vi "HTMLPlot_Create.vi"(0 "reference in":refnum<class "HTMLPlot.lvclass">, 1 "GraphContainer":refnum<k7>, 5 "error in (no error)":errorcluster, 6 "PlotType":T1) -> (14 "reference out":refnum<class "HTMLPlot.lvclass">, 19 "error out":errorcluster)   [LabVIEW 2019, in "HTMLPlot.lvclass"]
uses:
  HTMLPlot.lvclass
  <vilib>/numeric/Random Number (Range) U64.vi
  Controls/PlotType.ctl
panel:
  out "ReadyState":i32(ring)=4 items=["READYSTATE_UNINITIALIZED", "READYSTATE_LOADING", "READYSTATE_LOADED", "READYSTATE_INTERACTIVE", "READYSTATE_COMPLETE"]
  out "Get Reqest":string
  out "concatenated string":string
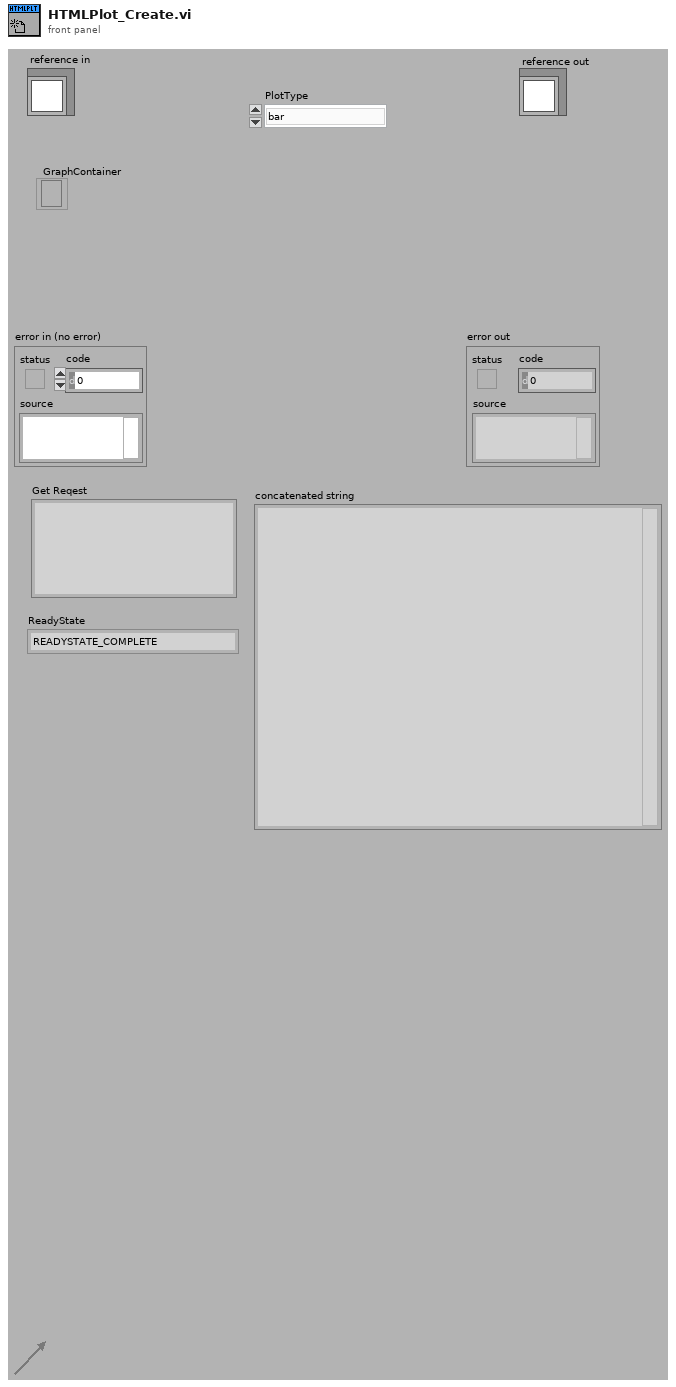
[diagram p1: front panel]
types:
  T1 = typedef "HTMLPlot.lvclass/PlotType.ctl" = enum16{"bar", "line", "pie"}
  T2 = enum16{"Standard", "Buffered", "CRLF", "Immediate"}
  T3 = typedef "HTMLPlot.lvclass/ObjectAttributes.ctl" = cluster{"Attribute1":dbl, "GraphContainer":refnum<k7>, "ChartScriptFile":string, "UtilScriptFile(demoData)":string, "BaseHTML":string, "GenericProperties":cluster{"PlotType":T1, "PlotTitle":string, "XLabel":string, "YLabel":string, "ShowToolTip":bool}, "LegendProperties":cluster{"Show":bool, "Position":T4}, "BarPlot":cluster{"Dataset":dbl[][], "DatasetLabels":string[], "XLabels":string[], "PlotColours":u32[], "Stacked":bool}, "PiePlot":cluster{"Dataset":dbl[][], "DatasetLabels":string[], "PlotColours":u32[], "DoughnutStyle":bool, "PlotLabels":string[]}, "connection ID":refnum<k5>, "PortID":u64}
  T4 = typedef "HTMLPlot.lvclass/LegendPosition.ctl" = enum16{"top", "right", "left", "bottom"}
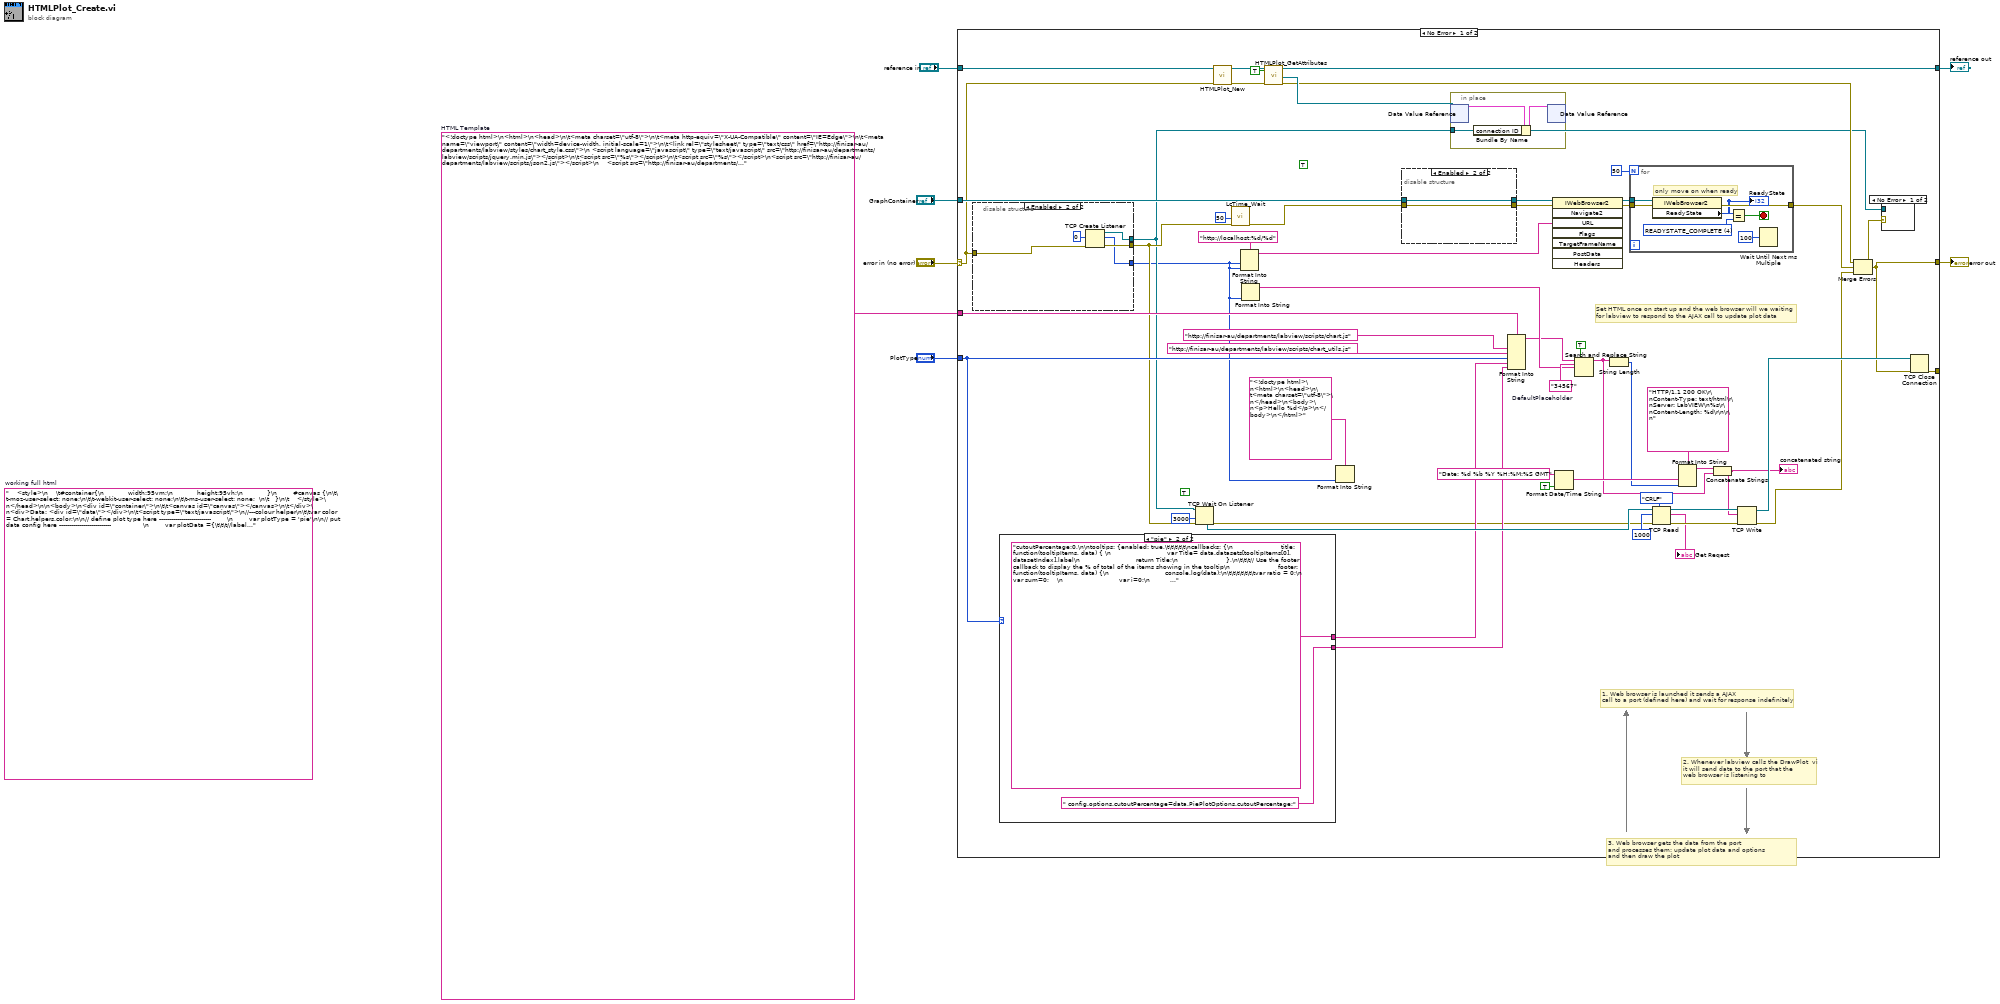
[diagram p0: block diagram]
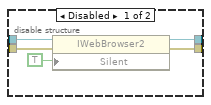
[diagram p2: hidden frame]
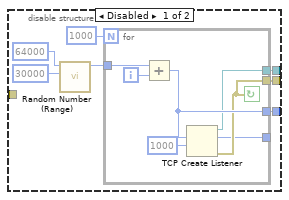
[diagram p3: hidden frame]
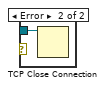
[diagram p4: hidden frame]
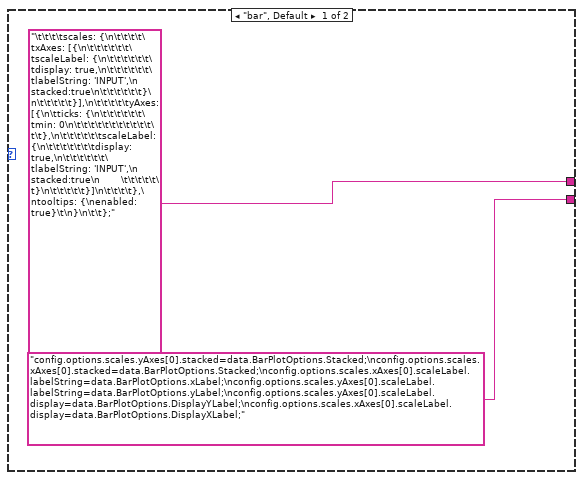
[diagram p5: hidden frame]
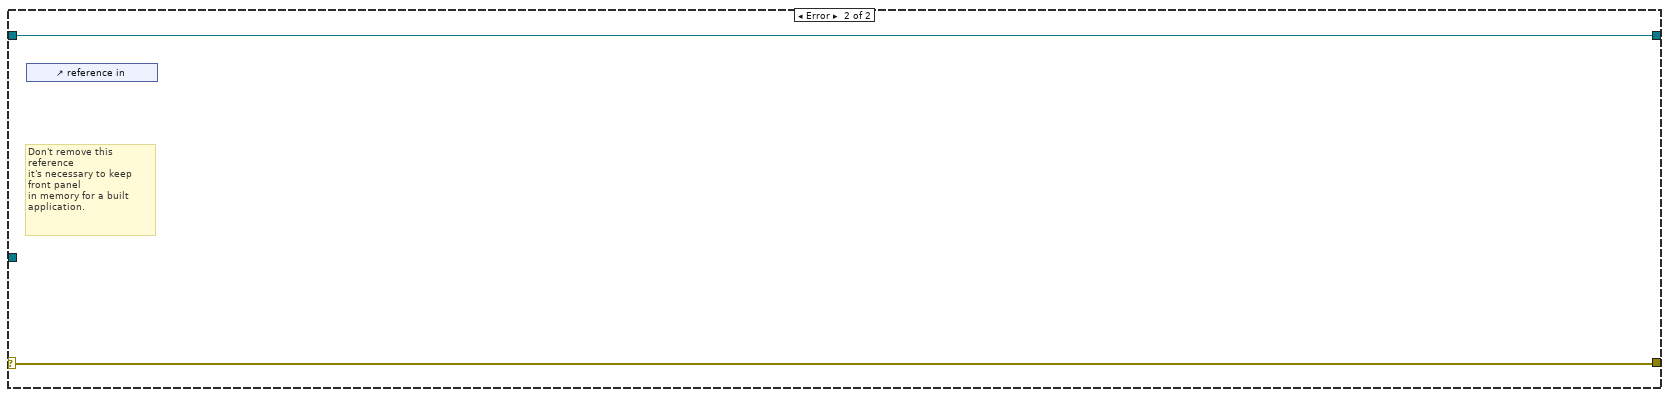
[diagram p6: hidden frame]
diagram:
  (unwired) "    <style>\n    \t#container{\n            width:95vm;\n            height:95vh;\n            }\n        #canvas {\n\t\t-moz-user-select: none;\n\t\t-webkit-user-select: none;\n\t\t-ms-user-select: none;  \n\t   }\n\t    </style>\n</head>\n\n<body>\n<div id=\"container\">\n\t\t<canvas id=\"canvas\"></canvas>\n\t</div>\n<div>Data: <div id=\"data\"></div>\n\t<script type=\"text/javascript\">\n//---colour helper\n\t\tvar color = Chart.helpers.color;\n\n// define plot type here --------------------------        \n        var plotType = 'pie'\n\n// put data config here --------------------------                \n        var plotData ={\t\t\t//labels\n   \tlabels: ['DLP2','SLP','DWP','DLP3'\n],\n    //datasets\n   datasets:[{\n\t\t\t\tlabel: 'Q1',\n\t\t\t\tbackgroundColor: ['#5C8260','#FF88C2','#2400B4','#FFF242'\n],\n\t\t\t\tdata: [3.000000,5.000000,7.000000,89.000000\n]\n\t\t\t},{\n\t\t\t\tlabel: 'Q2',\n\t\t\t\tbackgroundColor: ['#5C8260','#FF88C2','#2400B4','#FFF242'\n],\n\t\t\t\tdata: [2.000000,9.000000,3.000000,6.000000\n]\n\t\t\t}]}   \n// put plot options here --------------------------\n        var plotOptions ={responsive: true,\nmaintainAspectRatio: false,\n\t\t\t\tanimation: {\n\t\t\t\t\tanimateScale: true,\n\t\t\t\t\tanimateRotate: true\n\t\t\t\t},\nlegend: {\ndisplay:true,\t\t\t\t\t\t\nposition: 'right'\n\t\t\t\t\t},title: {\n\t\t\t\t\t\tdisplay:true,\n\t\t\t\t\t\ttext: 'Prouduction Summary 2020'\n\t\t\t\t\t}, tooltips: {enabled: true,\t\t\t\t\tcallbacks: {\n                        title: function(tooltipItems, data) { \n                            //console.log(data);\n                        var Title= data.datasets[tooltipItems[0].datasetIndex].label\n                            return Title;\n                        },\n\t\t\t// Use the footer callback to display the % of total of the items showing in the tooltip\n                        footer: function(tooltipItems, data) {\n                            console.log(data);\n\t\t\t\t\t\t\tvar ratio = 0;\n                            var sum=0;    \n                            var i=0;\n                            var length = data.datasets[tooltipItems[0].datasetIndex].data.length;\n                            for( i=0;i<length;i++){\n                                sum+= data.datasets[tooltipItems[0].datasetIndex].data[i];\n                            }\n\t\t\t\t\t\t\ttooltipItems.forEach(function(tooltipItem) {\n\t\t\t\t\t\t\t\tratio = 100*data.datasets[tooltipItem.datasetIndex].data[tooltipItem.index]/sum;\n                                ratio=ratio.toFixed(1)\n\t\t\t\t\t\t\t});\n\t\t\t\t\t\t\treturn 'ratio: ' + ratio + '%' ;\n\t\t\t\t\t\t},\n\t\t\t\t\t},\n\t\t\t\t\tfooterFontStyle: 'normal'}\t}\n // summarise config here --------------------------                   \n        var config = {\n\t\t\ttype: plotType,\n\t\t\tdata: plotData,\n\t\t\toptions: plotOptions\n\t\t};\n\n// run plot function here -------------------------- \n        \n\t\twindow.onload = function() {\n\t\t\tvar ctx = document.getElementById('canvas').getContext('2d');\n\t\t\twindow.myChart = new Chart(ctx, config); \n   CheckForEvents();\n\t\t};\n\nfunction CheckForEvents() {        \n        $.ajax({\n            url:'http://localhost:34567/action',\n             method:'GET',\n             dataType:'json',\n       \n            success: function(data){\n            config.type=data.data.PlotType;\n $(\"#data\").text(data.data.PlotData);\n console.log(data.data.PlotData);\nvar myObj = JSON.parse(data.data.PlotData);\n            config.data=myObj;\n console.log(myObj);\n//config.options=data.data.Options;\n          \n          window.myChart.update(); \n            CheckForEvents();\n            }\n        })\n     }\n\t</script>\n</body>\n</html>"  # working full html
  w2 = "<!doctype html>\n<html>\n<head>\n\t<meta charset=\"utf-8\">\n\t<meta http-equiv=\"X-UA-Compatible\" content=\"IE=Edge\">\n\t<meta name=\"viewport\" content=\"width=device-width, initial-scale=1\">\n\t<link rel=\"stylesheet\" type=\"text/css\" href=\"http://finisar-au/departments/labview/styles/chart_style.css\">\n <script language=\"javascript\" type=\"text/javascript\" src=\"http://finisar-au/departments/labview/scripts/jquery.min.js\"></script>\n\t<script src=\"%s\"></script>\n\t<script src=\"%s\"></script>\n<script src=\"http://finisar-au/departments/labview/scripts/json2.js\"></script>\n    <script src=\"http://finisar-au/departments/labview/scripts/jquery(v1.11.3).min.js\"></script>\n    <style>\n    \t#container{\n            width:95vm;\n            height:95vh;\n            }\n        #canvas {\n\t\t-moz-user-select: none;\n\t\t-webkit-user-select: none;\n\t\t-ms-user-select: none;  \n\t   }\n\t    </style>\n</head>\n\n<body>\n<div id=\"container\">\n\t\t<canvas id=\"canvas\"></canvas>\n\t</div>\n\t<script type=\"text/javascript\">\n//---colour helper\nvar color = Chart.helpers.color;\nvar plotData ={}  \n\n // summarise config here --------------------------                   \n        var config = {\n\n// **************** PLOT TYPE***************************\n\t\t\ttype: '%s',\n\n\t\t\tdata: plotData,\n//\t\t\t **************** PLOT OPTIONS : THIS PART WILL BE PLOT TYPE DEPENDENT***************************\noptions: \n{\nresponsive: true,\nmaintainAspectRatio: false,\n\t\t\t\tanimation: {\n\t\t\t\t\tanimateScale: true,\n\t\t\t\t\tanimateRotate: true\n\t\t\t\t},\nlegend: {\ndisplay:false,\t\t\t\t\t\t\nposition: 'right'\n\t\t\t\t\t},\ntitle: {\n\t\t\t\t\t\tdisplay:true,\n\t\t\t\t\t\ttext: 'INPUT'\n\t\t\t\t\t},  \n//*************************  ADDITIONAL OPTIONS   ***********************\n%s\n\n// run plot function here -------------------------- \n        \n\t\twindow.onload = function() {\n\t  var ctx = document.getElementById('canvas').getContext('2d');\n\t\t\twindow.myChart = new Chart(ctx, config); \n   CheckForEvents();\n\t\t};\n\nfunction CheckForEvents() {        \n        $.ajax({\n            url:'http://localhost:34567/action',\n             method:'GET',\n             dataType:'json',\n       \n            success: function(data){\n            var myData = JSON.parse(data.PlotData);\n            config.data=myData;\n\n            config.options.legend.display= data.GenericPlotOptions.LegendDisplay;\n            config.options.legend.position=data.GenericPlotOptions.LegendPosition;            \n           config.options.title.text=data.GenericPlotOptions.GraphTitle;\n\n//*************************  ADDITIONAL OPTIONS UPDATE ***********************\n%s\n\n//*************************  UPDATE PLOT ***********************\nwindow.myChart.update();\n\n//*************************  WAIT FOR UPDATE EVENT ***********************\nCheckForEvents();\n            }\n        })\n     }\n\t</script>\n</body>\n</html>"  # HTML Template
  n1 = case shown="No Error" "error in (no error)" {
    selector: "error in (no error)" -> [w16 w103]
    tunnel: [w25 w103] -> w7
    tunnel: "reference in" -> [w59 w102]
    tunnel: [w60 w102] -> w5
    tunnel: "GraphContainer" -> [w40 _]
    tunnel: "PlotType" -> [w36 _]
    tunnel: w2 -> [w54 _]
    tunnel: [w27 _] -> _
    frame No Error {
      (unwired) TRUE ("resolve remote address (T)")
      (unwired) TRUE
      w53 = "34567"  # DefaultPlaceholder
      # "3. Web browser gets the data from the port\nand processes them: update plot data and options\nand then draw the plot"
      # "2. Whenever labview calls the DrawPlot  vi \nit will send data to the port that the\nweb browser is listening to"
      # "1. Web browser is launched it sends a AJAX \ncall to a port (defined here) and wait for response indefinitely"
      # "Set HTML once on start up and the web browser will we waiting\nfor labview to respond to the AJAX call to update plot data"
      n2 = disable-structure shown="Enabled" {
        disable-tunnel: [w77 w92] -> w32
        disable-tunnel: [w76 w91] -> w24
        disable-tunnel: [w75 w90] -> w8
        disable-tunnel: w16 -> [_ w93]
        frame Disabled {
          n3 = call-poly <vilib>:"Random Number (Range).vi"("lower bound (0)"=u64 30000, "upper bound (100)"=u64 64000) -> ("number"=w79:u64)  [unwired: 9 in]
          n4 = for {
            N: 1000 -> [_]
            tunnel: [w83] -> w76
            tunnel: [w84] -> w77
            tunnel: w79 -> [w88]
            tunnel: [w86] -> w75
            tunnel: [w82] -> _
            i -> [w87]
            stop <- w84 continue-if-true
            n5 = Add(x=w88, y=w87) -> (x+y=w86:u64)
            n6 = TCP Create Listener(9:1000 ("timeout ms (25000)"), 10:w86) -> (0:w84:errorcluster, 2:w82:u16, 3:w83:refnum<k5>)  [unwired: 3 in]
          }
        }
        frame Enabled {
          n7 = TCP Create Listener(8:w93, 10:u16 0 ("port")) -> (0:w92:errorcluster, 2:w90:u16, 3:w91:refnum<k5>)  [unwired: 2 in, 1 out]
        }
      }
      n8 = case shown="\"pie\"" w36 {
        tunnel: ["\t\t\t\tscales: {\n\t\t\t\t\txAxes: [{\n\t\t\t\t\t\t\tscaleLabel: {\n\t\t\t\t\t\t\tdisplay: true,\n\t\t\t\t\t\t\tlabelString: 'INPUT',\n       stacked:true\n\t\t\t\t\t\t}\n\t\t\t\t\t}],\n\t\t\t\t\tyAxes: [{\n\tticks: {\n\t\t\t\t\t\t\tmin: 0\n\t\t\t\t\t\t\t\t\t\t\t\t\t},\n\t\t\t\t\t\tscaleLabel: {\n\t\t\t\t\t\t\tdisplay: true,\n\t\t\t\t\t\t\tlabelString: 'INPUT',\n       stacked:true\n       \t\t\t\t\t\t}\n\t\t\t\t\t}]\n\t\t\t\t},\ntooltips: {\nenabled: true}\t\n}\n\t\t};" "cutoutPercentage:0,\n\ntooltips: {enabled: true,\t\t\t\t\t\ncallbacks: {\n                        title: function(tooltipItems, data) { \n                            var Title= data.datasets[tooltipItems[0].datasetIndex].label\n                            return Title;\n                        },\n\t\t\t// Use the footer callback to display the % of total of the items showing in the tooltip\n                        footer: function(tooltipItems, data) {\n                            console.log(data);\n\t\t\t\t\t\t\tvar ratio = 0;\n                            var sum=0;    \n                            var i=0;\n                            var length = data.datasets[tooltipItems[0].datasetIndex].data.length;\n                            for( i=0;i<length;i++){\n                                sum+= data.datasets[tooltipItems[0].datasetIndex].data[i];\n                            }\n\t\t\t\t\t\t\ttooltipItems.forEach(function(tooltipItem) {\n\t\t\t\t\t\t\t\tratio = 100*data.datasets[tooltipItem.datasetIndex].data[tooltipItem.index]/sum;\n                                ratio=ratio.toFixed(1)\n\t\t\t\t\t\t\t});\n\t\t\t\t\t\t\treturn 'ratio: ' + ratio + '%' ;\n\t\t\t\t\t\t},\n\t\t\t\t\t},\n\t\t\t\t\tfooterFontStyle: 'normal'}\t}\n\t\t};"] -> w35
        tunnel: ["config.options.scales.yAxes[0].stacked=data.BarPlotOptions.Stacked;\nconfig.options.scales.xAxes[0].stacked=data.BarPlotOptions.Stacked;\nconfig.options.scales.xAxes[0].scaleLabel.labelString=data.BarPlotOptions.xLabel;\nconfig.options.scales.yAxes[0].scaleLabel.labelString=data.BarPlotOptions.yLabel;\nconfig.options.scales.yAxes[0].scaleLabel.display=data.BarPlotOptions.DisplayYLabel;\nconfig.options.scales.xAxes[0].scaleLabel.display=data.BarPlotOptions.DisplayXLabel;" " config.options.cutoutPercentage=data.PiePlotOptions.cutoutPercentage;"] -> w34
        frame "bar", Default {
        }
        frame "pie" {
        }
      }
      n9 = TCP Wait On Listener(8:w32, 9:3000 ("timeout ms (wait forever: -1)"), 11:w24) -> (0:w31:errorcluster, 4:w43:refnum<k5>)  [unwired: 1 in, 3 out]
      n10 = call "HTMLPlot_New.vi"("reference in"=w59, "error in (no error)"=w16) -> ("reference out"=w58:refnum<class "HTMLPlot.lvclass">, "error out"=w57:errorcluster)  [unwired: 14 in, 2 out]
      n11 = call "LcTime_Wait.vi"("msToWait"=u32 50, "error in (no error)"=w32) -> ("error out"=w30:errorcluster)  [unwired: 15 in, 2 out]
      n12 = Format Into String(format string="http://localhost:%d/%d", w8, w8) -> (resulting string=w49:string)  [unwired: 2 in, 1 out]
      n13 = Format Into String(w8) -> (resulting string=w51:string)  [unwired: 3 in, 1 out]
      n14 = call "HTMLPlot_GetAttributes.vi"("reference in"=w58, "OnlyGetDvrReference(False)"=TRUE, "error in (no error)"=w57) -> ("reference out"=w60:refnum<class "HTMLPlot.lvclass">, "DataRef"=w55:refnum<data-value>, "error out"=w41:errorcluster)  [unwired: 13 in, 1 out]
      n15 = Format Into String(format string="<!doctype html>\n<html>\n<head>\n\t<meta charset=\"utf-8\">\n</head>\n<body>\n<p>Hello %d</p>\n</body>\n</html>", w8) -> ()  [unwired: 2 in, 2 out]
      n16 = disable-structure shown="Enabled" {
        disable-tunnel: w40 -> [w65 w66]
        disable-tunnel: w30 -> [w64 w67]
        disable-tunnel: [w62 w66] -> w12
        disable-tunnel: [w61 w67] -> w11
        frame Disabled {
          n17 = property class="IWebBrowser2"(reference=w65, error in=w64, "Silent"=TRUE) -> (reference out=w62:refnum<k7>, error out=w61:errorcluster)
        }
        frame Enabled {
        }
      }
      n18 = in-place {
        in-place-border: w24 -> [w99]
        n19 = in-place-dvr #1(w55) -> (w101:T3)  [unwired: 1 out]
        n20 = Bundle By Name(cluster=w101, "connection ID"=w99) -> (w100:T3)
        n21 = in-place-dvr #1(w100) -> ()  [unwired: 2 out]
      }
      n22 = Format Into String(format string=w54, "http://finisar-au/departments/labview/scripts/chart.js" ("ChartScriptFile"), "http://finisar-au/departments/labview/scripts/chart_utils.js" ("UtilScriptFile(demoData)"), w36, w35, w34) -> (resulting string=w39:string)  [unwired: 2 in, 1 out]
      n23 = invoke class="IWebBrowser2" method="Navigate2"(reference=w12, error in=w11, "URL"=w49) -> (reference out=w14:refnum<k7>, error out=w13:errorcluster)  [unwired: 5 in, 6 out]
      n24 = Format Date/Time String(time format string (%c)="Date: %d %b %Y %H:%M:%S GMT", UTC format=TRUE) -> (date/time string=w20:string)  [unwired: 1 in]
      n25 = Search and Replace String(replace all?=TRUE ("replace all? (F)"), input string=w39, search string=w53, replace string=w51) -> (result string=w9:string)  [unwired: 4 in, 3 out]
      n26 = String Length(string=w9) -> (length=w19:i32)
      n27 = for {
        N: 50 -> [_]
        tunnel: w14 -> [w74]
        tunnel: w13 -> [w70]
        tunnel: [w69] -> w42
        stop <- w72 stop-if-true
        w73 = 4 items=["READYSTATE_UNINITIALIZED", "READYSTATE_LOADING", "READYSTATE_LOADED", "READYSTATE_INTERACTIVE", "READYSTATE_COMPLETE"] ("ReadyState")
        # "only move on when ready"
        n28 = property class="IWebBrowser2"(reference=w74, error in=w70) -> (error out=w69:errorcluster, "ReadyState"=w68:i32)  [unwired: 1 out]
        "ReadyState" <- w68
        n29 = Equal?(x=w68, y=w73) -> (x = y?=w72:bool)
        n30 = Wait Until Next ms Multiple(millisecond multiple=u32 100) -> ()  [unwired: 1 out]
      }
      n31 = TCP Read(connection ID=w43, bytes to read=1000, error in (no error)=w31, 7:T2."CRLF" ("mode (standard)")) -> (connection ID out=w46:refnum<k5>, data out=→"Get Reqest":string, error out=w45:errorcluster)  [unwired: 1 in]
      n32 = Format Into String(format string="HTTP/1.1 200 OK\r\nContent-Type: text/html\r\nServer: LabVIEW\n%s\r\nContent-Length: %d\r\n\r\n", w20, w19) -> (resulting string=w18:string)  [unwired: 2 in, 1 out]
      n33 = Concatenate Strings(w18, w9) -> (w17:string)
      "concatenated string" <- w17
      n34 = TCP Write(connection ID=w46, data in=w17, error in (no error)=w45) -> (connection ID out=w44:refnum<k5>, error out=w28:errorcluster)  [unwired: 1 in, 1 out]
      n35 = Merge Errors(w41, w42, w28) -> (w25:errorcluster)
      n36 = case shown="No Error" w25 {
        tunnel: w24 -> [_ w94]
        frame No Error {
        }
        frame Error {
          n37 = TCP Close Connection(connection ID=w94) -> ()  [unwired: 2 in, 2 out]
        }
      }
      n38 = TCP Close Connection(connection ID=w44, error in (no error)=w25) -> (error out=w27:errorcluster)  [unwired: 1 in, 1 out]
    }
    frame Error {
      # "Don't remove this reference\nit's necessary to keep front panel\nin memory for a built application."
      n39 = control-ref of="reference in"() -> ()  [unwired: 1 out]
    }
  }
  "error out" <- w7
  "reference out" <- w5
